vi "Regler darf starten.vi"(11 "Regler start":bool) -> (3 "Regler darf starten":bool)   [LabVIEW 2014]
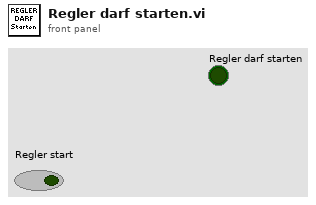
[diagram p1: front panel]
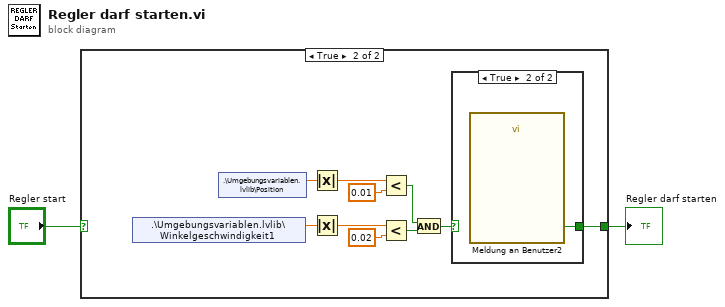
[diagram p0: block diagram]
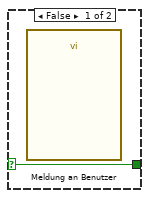
[diagram p3: hidden frame]
diagram:
  n1 = case shown="True" "Regler start" {
    selector: "Regler start" -> [w3 _]
    tunnel: [w3 w4] -> w1
    frame False {
    }
    frame True {
      n2 = shared-variable ".\\Umgebungsvariablen.lvlib\\Winkelgeschwindigkeit1"() -> (w10:dbl)  [unwired: 1 in, 1 out]
      n3 = shared-variable ".\\Umgebungsvariablen.lvlib\\Position"() -> (w12:dbl)  [unwired: 1 in, 1 out]
      n4 = Absolute Value(x=w12) -> (abs(x)=w13:dbl)
      n5 = Absolute Value(x=w10) -> (abs(x)=w9:dbl)
      n6 = Less?(x=w13, y=0.01) -> (x < y?=w6:bool)
      n7 = Less?(x=w9, y=0.02) -> (x < y?=w7:bool)
      n8 = And(x=w6, y=w7) -> (x .and. y?=w5:bool)
      n9 = case shown="True" w5 {
        selector: w5 -> [w14 _]
        tunnel: [w14 w15] -> w4
        frame False {
          n10 = call "Meldung an Benutzer"() -> ()  [unwired: 10 in, 2 out]
        }
        frame True {
          n11 = call "Meldung an Benutzer2"() -> ("OK"=w15:bool)  [unwired: 10 in, 1 out]
        }
      }
    }
  }
  "Regler darf starten" <- w1
